vi "Find_OriginalNameOfTemporaryFile.vi"(8 "error in (no error)":errorcluster, 10 "TempName":string="about: C:\\Users\\Marco Preziani\\AppData\\Local\\Temp\\lvtemp389.tmp\\criteria\\criteria_window.html\"", 11 "object in":refnum<class "Folder_Mgmt.lvclass">) -> (0 "error out":errorcluster, 1 "File":string, 2 "Folder":string, 3 "object out":refnum<class "Folder_Mgmt.lvclass">)   [LabVIEW 2016, in "Folder_Mgmt.lvclass"]
uses:
  Folder_Mgmt.lvclass
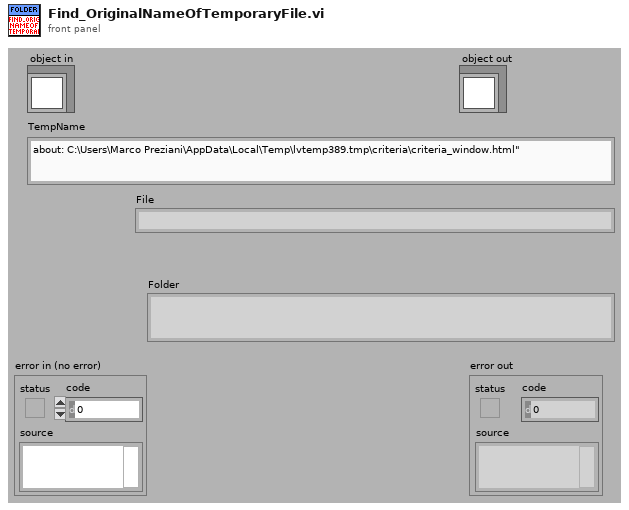
[diagram p1: front panel]
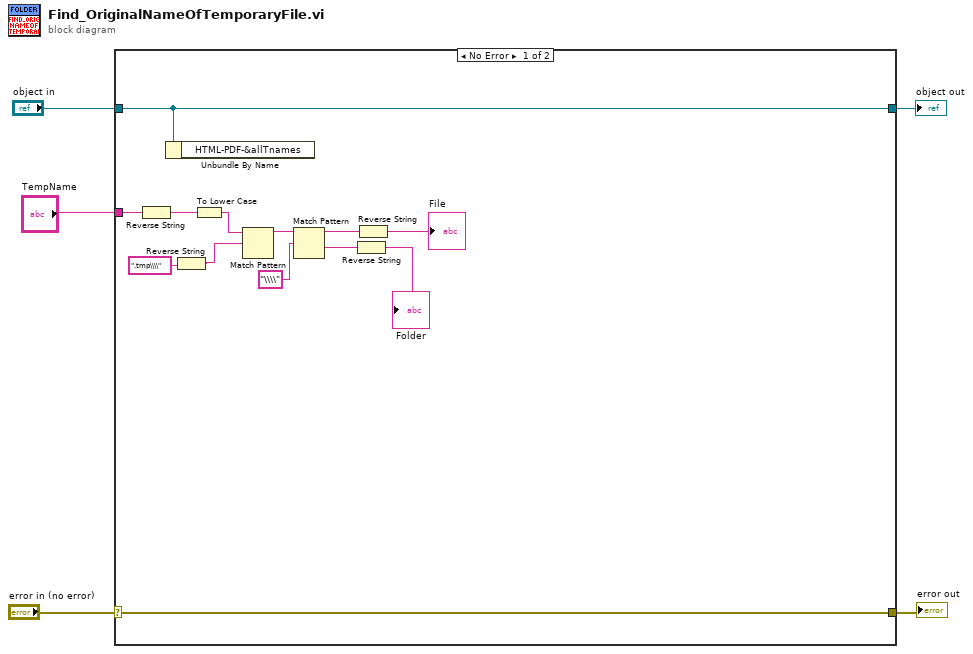
[diagram p0: block diagram]
diagram:
  n1 = case shown="No Error" "error in (no error)" {
    selector: "error in (no error)" -> [w18 w20]
    tunnel: [w18 w20] -> w4
    tunnel: [w17 w19] -> w2
    tunnel: "object in" -> [w17 w19]
    tunnel: "TempName" -> [w16 _]
    frame No Error {
      n2 = Reverse String(1:w16) -> (0:w15:string)
      n3 = Unbundle By Name(w17) -> ()  [unwired: 1 out]
      n4 = Reverse String(1:".tmp\\\\") -> (0:w12:string)
      n5 = To Lower Case(string=w15) -> (all lower case string=w13:string)
      n6 = Match Pattern(string=w13, regular expression=w12) -> (before substring=w11:string)  [unwired: 1 in, 3 out]
      n7 = Match Pattern(string=w11, regular expression="\\\\") -> (before substring=w9:string, after substring=w7:string)  [unwired: 1 in, 2 out]
      n8 = Reverse String(1:w7) -> (0:→"Folder":string)
      n9 = Reverse String(1:w9) -> (0:→"File":string)
    }
    frame Error {
    }
  }
  "error out" <- w4
  "object out" <- w2
